vi "filter_File.vi"() -> ()   [LabVIEW 2020]
uses:
  <vilib>/Utility/file.llb/Write Delimited Spreadsheet (string).vi
panel:
  in  "file path (dialog if empty)":path=path "C:/Users/jumpodp/Downloads/csv-20240610T071920Z-001/summary.csv"
  out "Array":string[][](array[string])
  out "All Files in Dir":path[](array[path])
  in  "Folder":path=path "C:/Users/jumpodp/Downloads/csv-20240610T071920Z-001/csv"
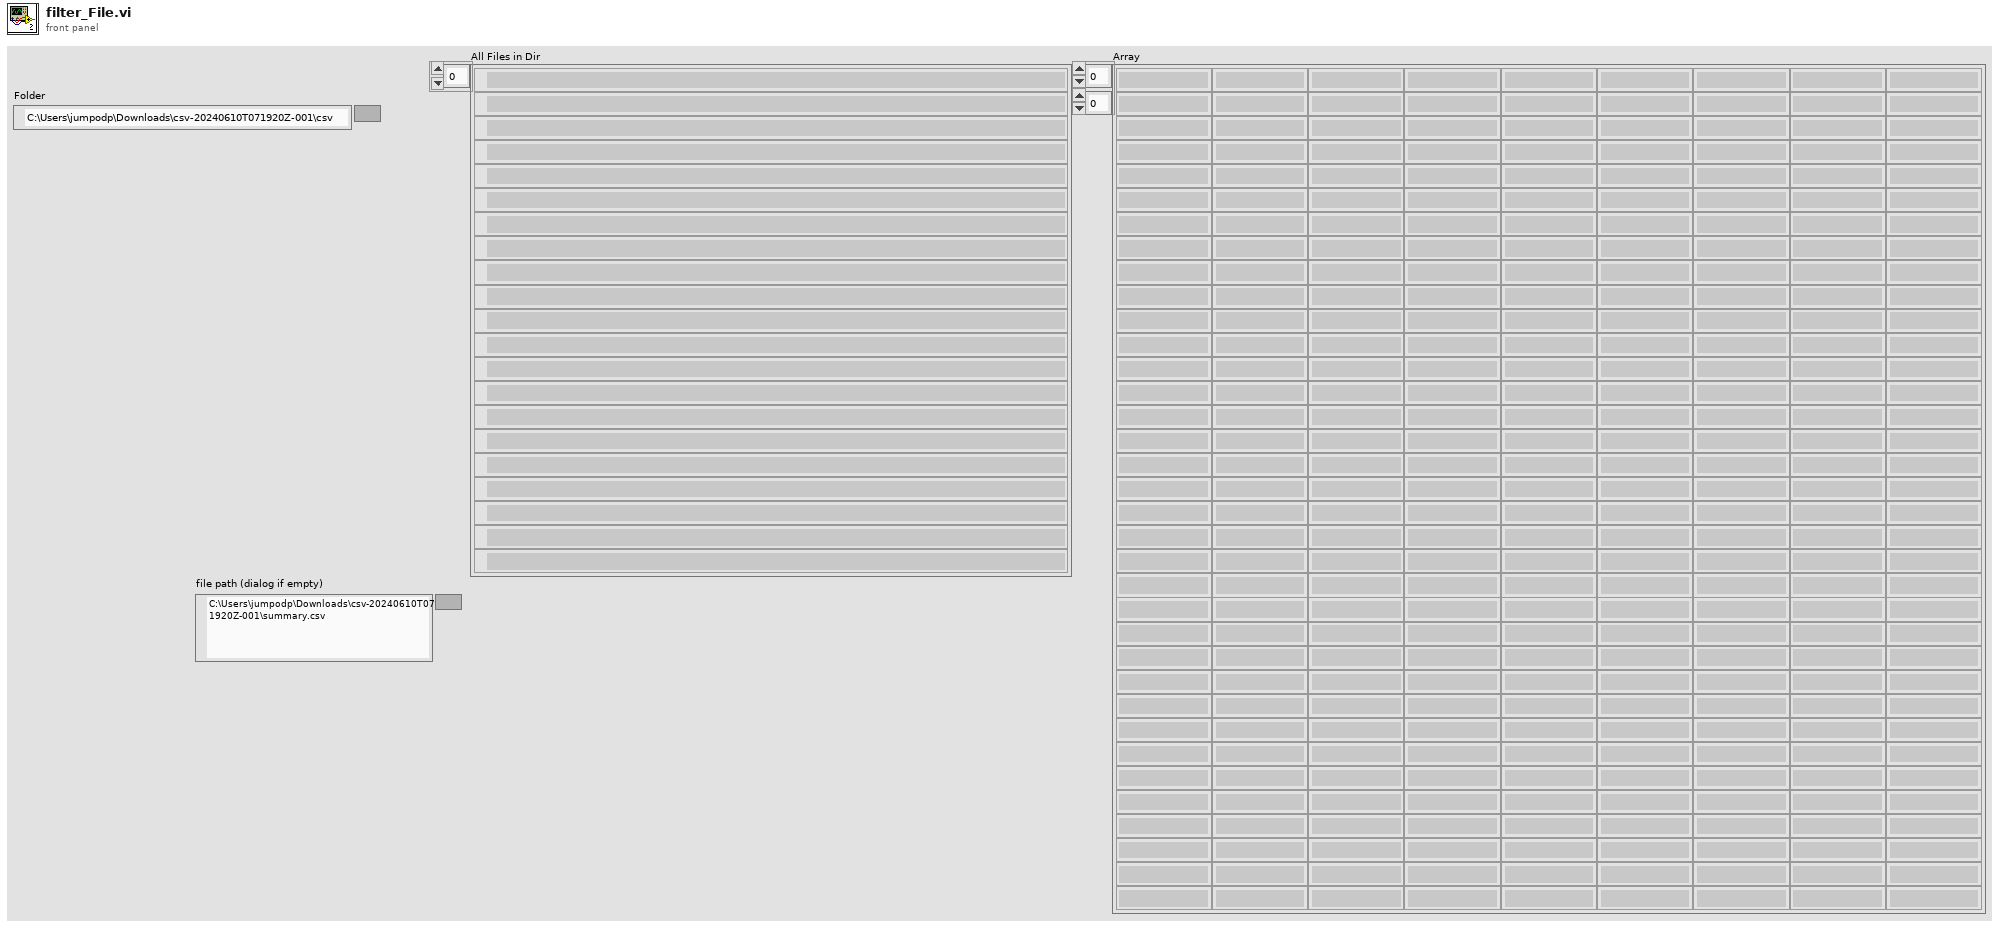
[diagram p1: front panel]
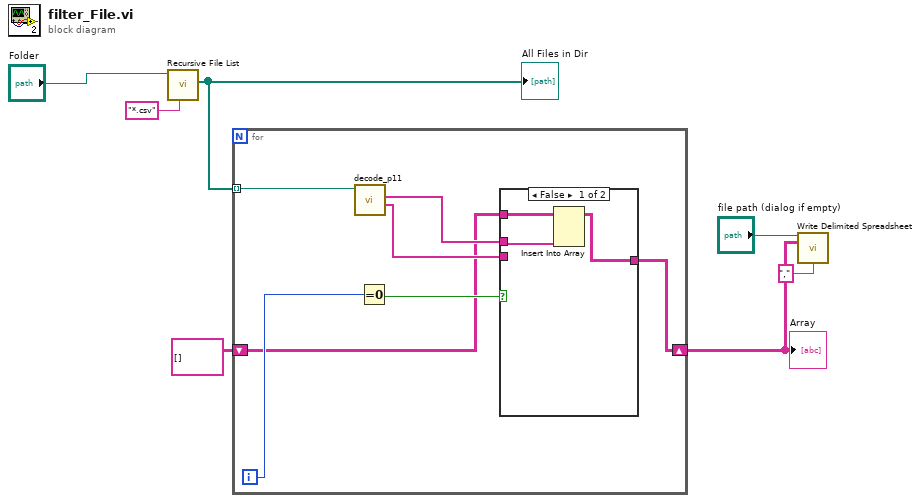
[diagram p0: block diagram]
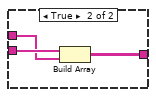
[diagram p2: hidden frame]
diagram:
  n1 = call <vilib>:"Recursive File List.vi"("pattern"="*.csv", "Folder Path"="Folder") -> ("All Files in Dir"=w5:path[])  [unwired: 5 in, 4 out]
  "All Files in Dir" <- w5
  n2 = for {
    tunnel: w5 -> [w14] mode=indexing
    shift-right: [w9] -> w3
    shift-left: string[][] [] -> [w8]
    i -> [w13]
    n3 = call "decode_p11.vi"("file path (dialog if empty)"=w14) -> ("HeadeR"=w11:string[], "Data"=w10:string[])  [unwired: 8 in, 1 out]
    n4 = Equal To 0?(x=w13) -> (x = 0?=w12:bool)
    n5 = case shown="False" w12 {
      tunnel: w11 -> [_ w20]
      tunnel: w10 -> [w15 w19]
      tunnel: [w16 w18] -> w9
      tunnel: w8 -> [w17 _]
      frame False {
        n6 = Insert Into Array(array=w17, new element=w15) -> (w16:string[][])  [unwired: 2 in]
      }
      frame True {
        n7 = Build Array(w20, w19) -> (w18:string[][])
      }
    }
  }
  "Array" <- w3
  n8 = call-poly <vilib>:"Write Delimited Spreadsheet.vi"("file path (dialog if empty)"="file path (dialog if empty)", "2D data"=w3, "delimiter (\\t)"="," ("delimiter (\\t)")) -> ()  [unwired: 11 in, 2 out]
